vi "Main.vi"() -> ()   [LabVIEW 2026]
doc: "This template is for the Queued Message Handler design pattern.\n\nThe Event Handling Loop generates messages based on user interface actions.\n\nThe Message Handling Loop processes messages generated by the Event Handling Loop, or by other messages. The messages are string values, so new messages can be added easily to the Message Cases case structure in the Message Handling Loop. Each message cluster can also provide an optional value for Message Data, which is a variant that can be converted to whatever message-specific data is required."
uses:
  controls/Controls.ctl
  controls/Program_Settings.ctl
  controls/Display_Panel.ctl
  controls/UI Data.ctl
  support/Message Queue/Enqueue Message (Single).vi
  <vilib>/Utility/error.llb/Error Cluster From Error Code.vi
  <vilib>/ErrorRing/Error Ring.xnode
  support/Message Queue/Message Queue.lvlib
  support/User Event - Stop/User Event - Stop.lvlib
panel:
  out "Display Panel":T1 {"Run time" format="%#_4g"}
  in  "Cluster":T2
  in  "Controls":T3 {"Incline" min=0.0 max=10.0 step=1.0 format="%#_2g"; "Speed" min=0.0 max=10.0 step=0.5 format="%#_2g"}
  in  "Exit":bool
  # "Control Panel"
  # "Manual Setting"
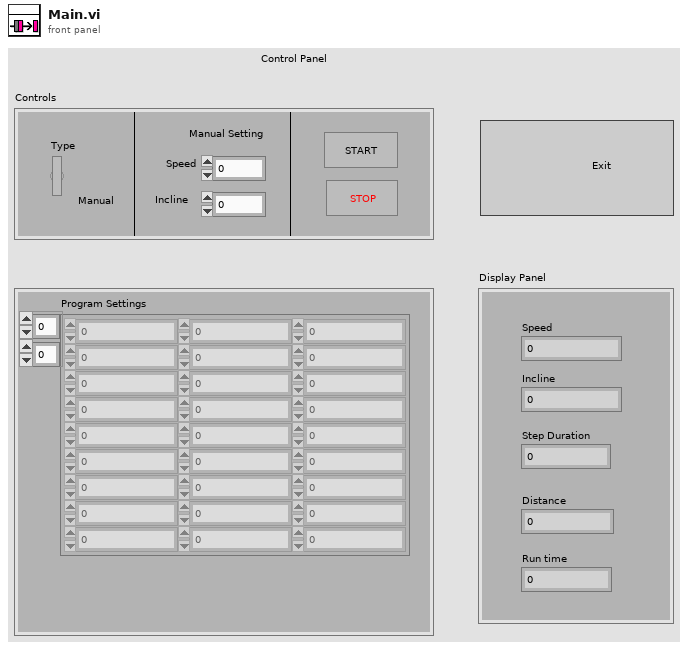
[diagram p1: front panel]
types:
  T1 = typedef "Display_Panel.ctl" = cluster{"Speed":dbl, "Incline":dbl, "Step Duration":dbl, "Distance":dbl, "Run time":dbl}
  T2 = typedef "Program_Settings.ctl" = cluster{"Program Settings":dbl[][]}
  T3 = typedef "Controls.ctl" = cluster{"Type":bool, "Speed":dbl, "Incline":dbl, "Start":bool, "stop":bool}
  T4 = typedef "UI Data.ctl" = cluster{"Boolean":bool, "String":string, "Tick Count":dbl, "Data Display Ref":refnum<vi>, "Exit Button Ref":refnum<vi>, "Display Panel":T1, "Controls":T3, "Controls Ref":refnum<vi>, "Display Panel Ref":refnum<vi>, "Tick Counter":dbl}
  T5 = typedef "Message Queue.lvlib/All Message Queues.ctl" = cluster{"UI":refnum<queue>}
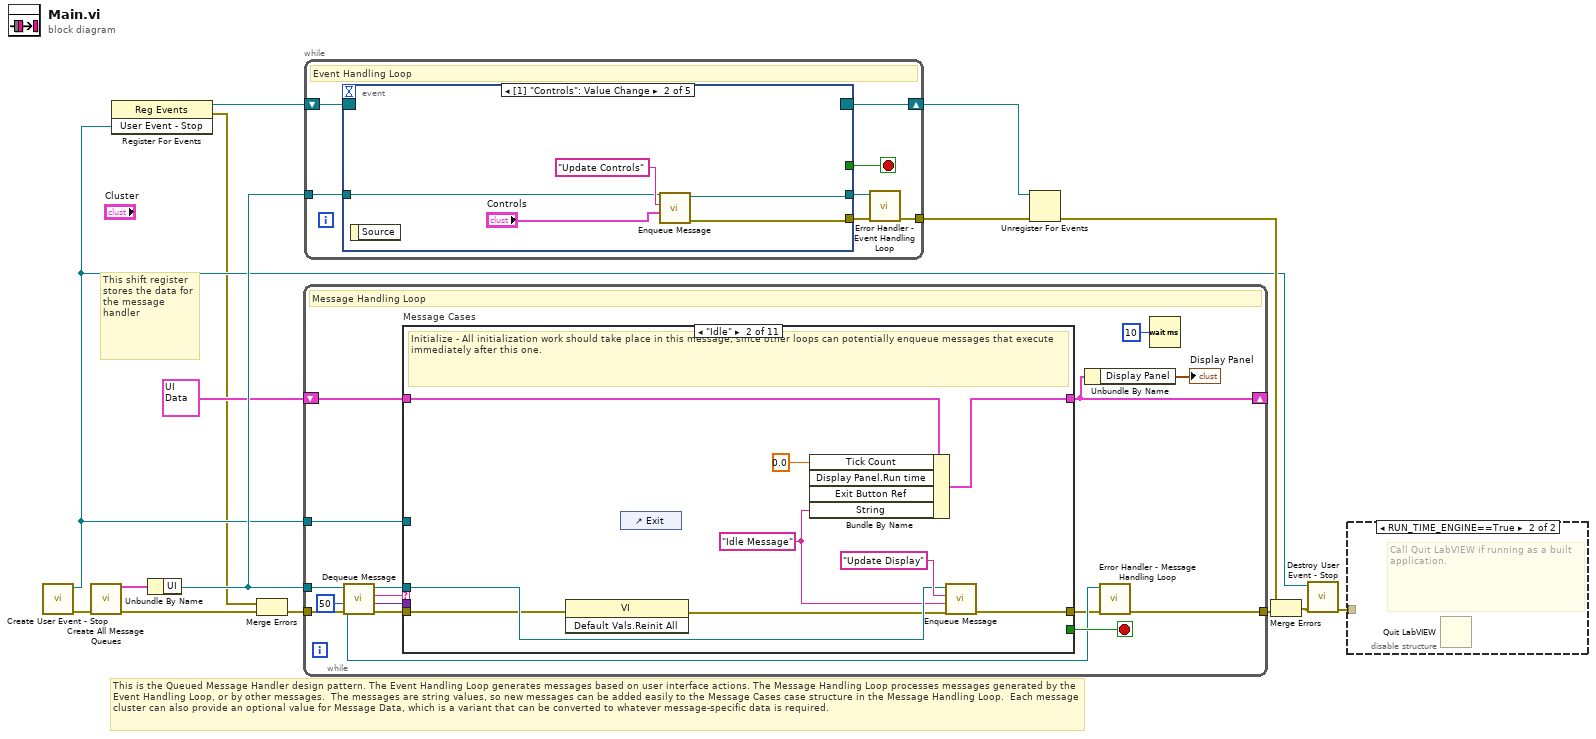
[diagram p0: block diagram]
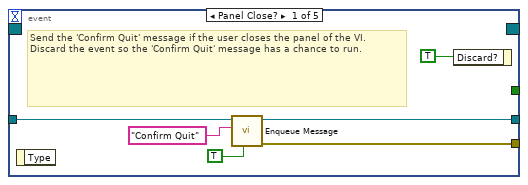
[diagram p3: hidden frame]
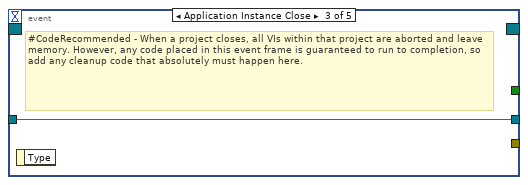
[diagram p4: hidden frame]
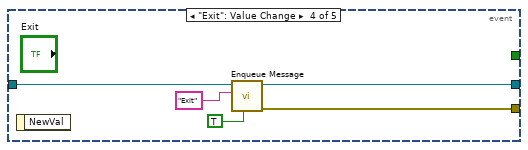
[diagram p5: hidden frame]
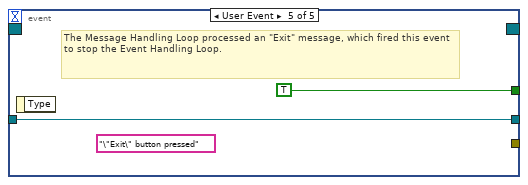
[diagram p6: hidden frame]
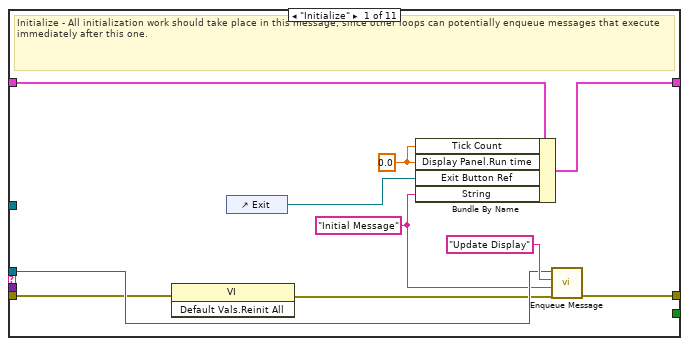
[diagram p7: hidden frame]
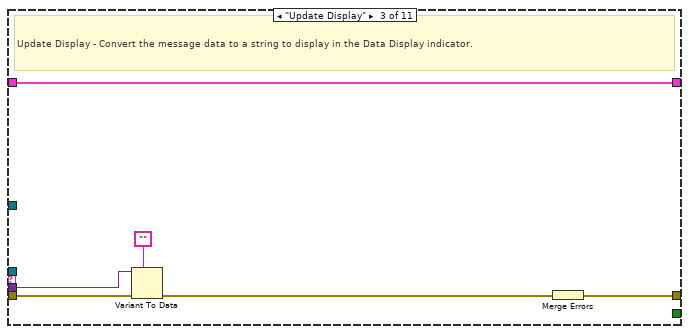
[diagram p8: hidden frame]
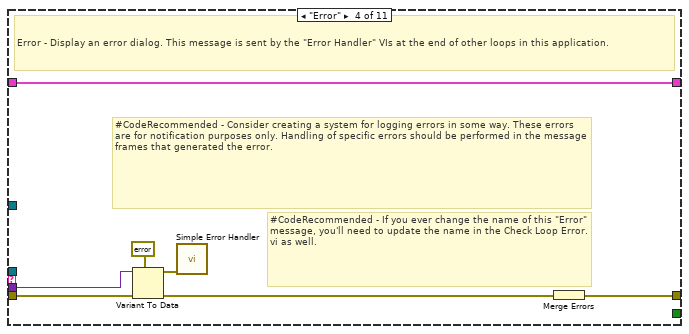
[diagram p9: hidden frame]
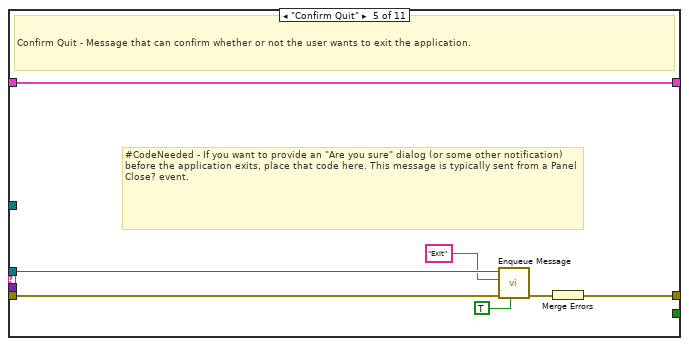
[diagram p10: hidden frame]
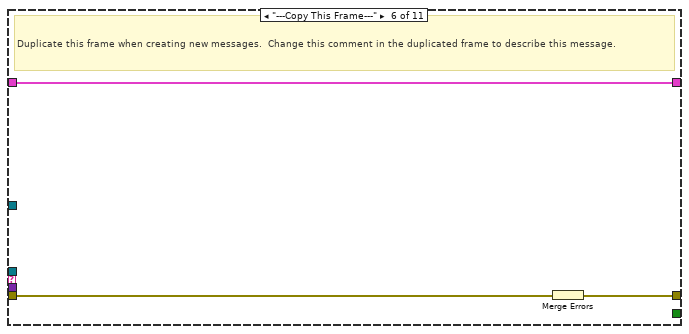
[diagram p11: hidden frame]
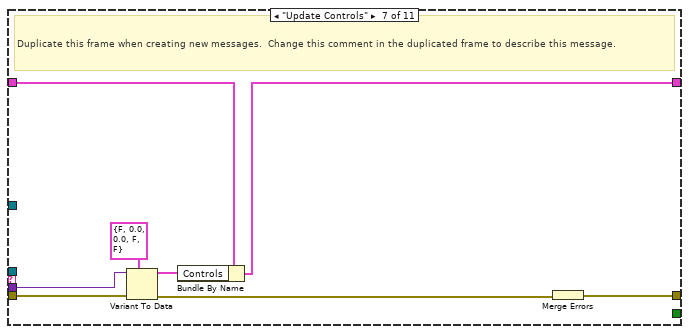
[diagram p12: hidden frame]
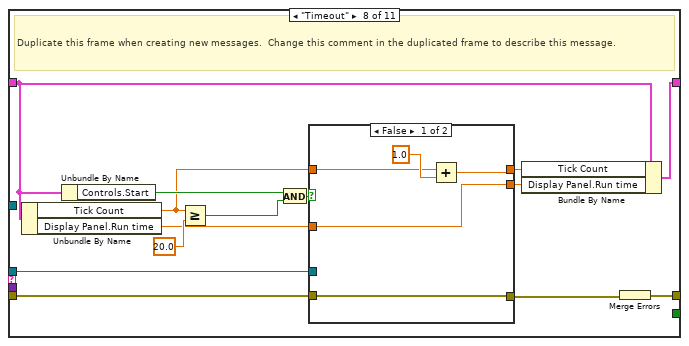
[diagram p13: hidden frame]
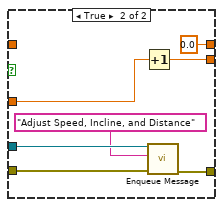
[diagram p14: hidden frame]
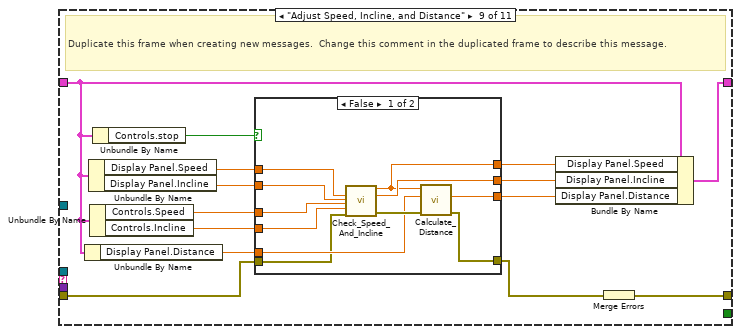
[diagram p15: hidden frame]
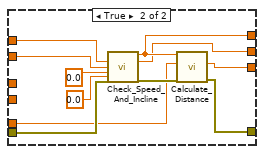
[diagram p16: hidden frame]
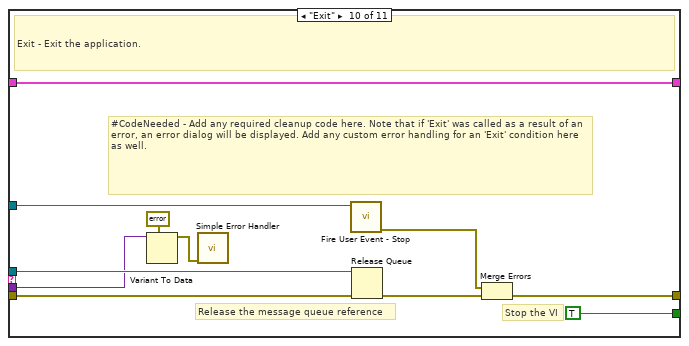
[diagram p17: hidden frame]
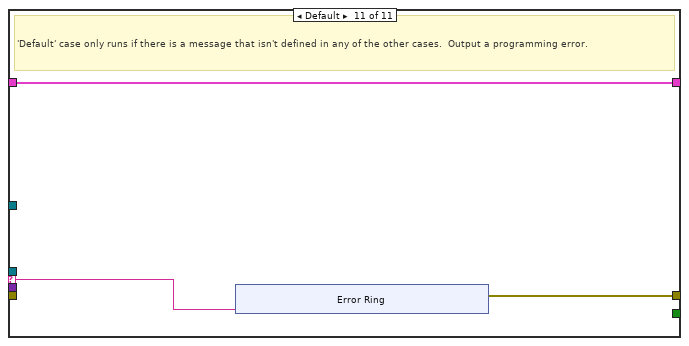
[diagram p18: hidden frame]
diagram:
  # "This is the Queued Message Handler design pattern. The Event Handling Loop generates messages based on user interface actions. The Message Handling Loop processes messages generated by the Event Handling Loop, or by other messages.  The messages are string values, so new messages can be added easily to the Message Cases case structure in the Message Handling Loop.  Each message cluster can also provide an optional value for Message Data, which is a variant that can be converted to whatever message-specific data is required."
  # "This shift register stores the data for the message handler"
  n1 = call "Create User Event - Stop.vi"() -> ("error out"=w11:errorcluster, "User Event - Stop"=w3:refnum<user-event>)  [unwired: 10 in]
  n2 = call "Create All Message Queues.vi"("error in (no error)"=w11) -> ("error out"=w15:errorcluster, "Message Queues out"=w14:T5)  [unwired: 9 in]
  n3 = register-events(w3) -> (reference out=w4:refnum<event-registration>, error out=w1:errorcluster)  [unwired: 2 in]
  n4 = Unbundle By Name(w14) -> ("UI"=w12:refnum<queue>)
  n5 = Merge Errors(w1, w15) -> (w2:errorcluster)
  n6 = while {
    tunnel: w12 -> [w23]
    shift-right: [w19] -> _
    shift-left: T4 {"Boolean"=FALSE, "String"="", "Tick Count"=0.0, "Data Display Ref"=refnum, "Exit Button Ref"=refnum, "Display Panel"={"Speed"=0.0, "Incline"=0.0, "Step Duration"=0.0, "Distance"=0.0, "Run time"=0.0}, "Controls"={"Type"=FALSE, "Speed"=0.0, "Incline"=0.0, "Start"=FALSE, "stop"=FALSE}, "Controls Ref"=refnum, "Display Panel Ref"=refnum, "Tick Counter"=0.0} ("Data Cluster") -> [w30]
    tunnel: w3 -> [w28]
    tunnel: w2 -> [w27]
    tunnel: [w21] -> w13
    stop <- w29 stop-if-true
    # "Message Handling Loop"
    n7 = call "Dequeue Message.vi"("error in (no error)"=w27, "timeout in ms (-1)"=50, "Message Queue"=w23) -> ("error out"=w26:errorcluster, "Message Data"=w24:variant, "Message"=w25:string, "dup Message Queue"=w22:refnum<queue>)  [unwired: 5 in]
    n8 = case "Message Cases" shown="\"Idle\"" w25 {
      selector: w25 -> [_ _ _ _ _ _ _ _ _ _ w154]
      tunnel: w22 -> [w35 w45 _ _ w65 _ _ w90 _ w153 _]
      tunnel: w26 -> [w33 w43 w53 w62 w69 w72 w79 w92 w113 w146 _]
      tunnel: [w40 w49 w54 w56 w67 w70 w80 w94 w120 w149 w155] -> w20
      tunnel: w30 -> [w39 w48 w55 w61 w68 w71 w75 w89 w109 w152 w156]
      tunnel: [w38 w47 w55 w61 w68 w71 w73 w93 w119 w152 w156] -> w19
      tunnel: [_ _ _ _ _ _ _ _ _ TRUE _] -> w29
      tunnel: w24 -> [_ _ w52 w60 _ _ w77 _ _ w143 _]
      tunnel: w28 -> [_ _ _ _ _ _ _ _ _ w148 _]
      frame "Initialize" {
        w31 = 0.0 ("Total Time")
        w34 = "Initial Message" ("Initial Message")
        # "Initialize - All initialization work should take place in this message, since other loops can potentially enqueue messages that execute immediately after this one."
        n9 = invoke class="VI" method="Default Vals.Reinit All"(error in=w33) -> (error out=w32:errorcluster)  [unwired: 2 in, 2 out]
        n10 = control-ref of="Exit"() -> (w37:refnum<vi>)
        n11 = Bundle By Name(cluster=w39, "Tick Count"=w31, "Display Panel.Run time"=w31, "Exit Button Ref"=w37, "String"=w34) -> (w38:T4)
        n12 = call-poly "Enqueue Message.vi"("error in (no error)"=w32, "Message Data"=w34, "Message"="Update Display", "Message Queue"=w35) -> ("error out"=w40:errorcluster)  [unwired: 6 in, 1 out]
      }
      frame "Idle" {
        w44 = "Idle Message" ("Initial Message")
        # "Initialize - All initialization work should take place in this message, since other loops can potentially enqueue messages that execute immediately after this one."
        n13 = invoke class="VI" method="Default Vals.Reinit All"(error in=w43) -> (error out=w42:errorcluster)  [unwired: 2 in, 2 out]
        n14 = control-ref of="Exit"() -> ()  [unwired: 1 out]
        n15 = Bundle By Name(cluster=w48, "Tick Count"=0.0 ("Total Time"), "String"=w44) -> (w47:T4)  [unwired: 2 in]
        n16 = call-poly "Enqueue Message.vi"("error in (no error)"=w42, "Message Data"=w44, "Message"="Update Display", "Message Queue"=w45) -> ("error out"=w49:errorcluster)  [unwired: 6 in, 1 out]
      }
      frame "Update Display" {
        # "Update Display - Convert the message data to a string to display in the Data Display indicator."
        n17 = Variant To Data(error in=w53, type="", Variant=w52) -> (error out=w50:errorcluster)  [unwired: 1 out]
        n18 = Merge Errors(w50) -> (w54:errorcluster)
      }
      frame "Error" {
        # "#CodeRecommended - If you ever change the name of this \"Error\" message, you'll need to update the name in the Check Loop Error.vi as well."
        # "#CodeRecommended - Consider creating a system for logging errors in some way. These errors are for notification purposes only. Handling of specific errors should be performed in the message frames that generated the error."
        # "Error - Display an error dialog. This message is sent by the \"Error Handler\" VIs at the end of other loops in this application."
        n19 = Variant To Data(error in=w62, type=errorcluster {"status"=FALSE, "code"=0, "source"=""} ("error constant"), Variant=w60) -> (data=w58:errorcluster, error out=w57:errorcluster)
        n20 = call <vilib>:"Simple Error Handler.vi"("error in (no error)"=w58) -> ()  [unwired: 4 in, 5 out]
        n21 = Merge Errors(w57) -> (w56:errorcluster)
      }
      frame "Confirm Quit" {
        # "#CodeNeeded - If you want to provide an \"Are you sure\" dialog (or some other notification) before the application exits, place that code here. This message is typically sent from a Panel Close? event."
        # "Confirm Quit - Message that can confirm whether or not the user wants to exit the application."
        n22 = call-poly "Enqueue Message.vi"("Priority Message? (F)"=TRUE, "error in (no error)"=w69, "Message"="Exit", "Message Queue"=w65) -> ("error out"=w66:errorcluster)  [unwired: 6 in, 1 out]
        n23 = Merge Errors(w66) -> (w67:errorcluster)
      }
      frame "---Copy This Frame---" {
        # "Duplicate this frame when creating new messages.  Change this comment in the duplicated frame to describe this message."
        n24 = Merge Errors(w72) -> (w70:errorcluster)
      }
      frame "Update Controls" {
        # "Duplicate this frame when creating new messages.  Change this comment in the duplicated frame to describe this message."
        n25 = Variant To Data(error in=w79, type=T3 {"Type"=FALSE, "Speed"=0.0, "Incline"=0.0, "Start"=FALSE, "stop"=FALSE} ("Controls"), Variant=w77) -> (data=w74:T3, error out=w78:errorcluster)
        n26 = Bundle By Name(cluster=w75, "Controls"=w74) -> (w73:T4)
        n27 = Merge Errors(w78) -> (w80:errorcluster)
      }
      frame "Timeout" {
        # "Duplicate this frame when creating new messages.  Change this comment in the duplicated frame to describe this message."
        n28 = Unbundle By Name(w89) -> ("Tick Count"=w84:dbl, "Display Panel.Run time"=w81:dbl)
        n29 = Unbundle By Name(w89) -> ("Controls.Start"=w88:bool)
        n30 = Greater Or Equal?(x=w84, y=20.0) -> (x >= y?=w82:bool)
        n31 = And(x=w88, y=w82) -> (x .and. y?=w87:bool)
        n32 = case shown="False" w87 {
          tunnel: w92 -> [w99 w106]
          tunnel: [w99 w105] -> w91
          tunnel: w90 -> [_ w104]
          tunnel: w84 -> [w96 _]
          tunnel: [w95 w101] -> w86
          tunnel: [w97 0.0] -> w85
          tunnel: w81 -> [w95 w100]
          frame False {
            n33 = Add(x=w96, y=1.0) -> (x+y=w97:dbl)
          }
          frame True {
            n34 = Increment(x=w100) -> (x+1=w101:dbl)
            n35 = call-poly "Enqueue Message.vi"("error in (no error)"=w106, "Message"="Adjust Speed, Incline, and Distance", "Message Queue"=w104) -> ("error out"=w105:errorcluster)  [unwired: 7 in, 1 out]
          }
        }
        n36 = Bundle By Name(cluster=w89, "Tick Count"=w85, "Display Panel.Run time"=w86) -> (w93:T4)
        n37 = Merge Errors(w91) -> (w94:errorcluster)
      }
      frame "Adjust Speed, Incline, and Distance" {
        # "Duplicate this frame when creating new messages.  Change this comment in the duplicated frame to describe this message."
        n38 = Unbundle By Name(w109) -> ("Display Panel.Distance"=w112:dbl)
        n39 = Unbundle By Name(w109) -> ("Display Panel.Speed"=w116:dbl, "Display Panel.Incline"=w118:dbl)
        n40 = Unbundle By Name(w109) -> ("Controls.Speed"=w111:dbl, "Controls.Incline"=w117:dbl)
        n41 = Unbundle By Name(w109) -> ("Controls.stop"=w108:bool)
        n42 = case shown="False" w108 {
          tunnel: w118 -> [w131 w139]
          tunnel: w117 -> [w130 _]
          tunnel: w116 -> [w122 w138]
          tunnel: [w121 w133] -> w115
          tunnel: [w129 w132] -> w114
          tunnel: w113 -> [w124 w142]
          tunnel: w112 -> [w127 w134]
          tunnel: w111 -> [w126 _]
          tunnel: [w125 w135] -> w110
          tunnel: [w123 w136] -> w107
          frame False {
            n43 = call "Check_Speed_And_Incline.vi"("Display Speed"=w122, "Display Incline"=w131, "Control Speed"=w126, "Control Incline"=w130, "error in (no error)"=w124) -> ("Speed"=w121:dbl, "Incline"=w129:dbl, "error out"=w128:errorcluster)  [unwired: 8 in]
            n44 = call "Calculate_Distance.vi"("Speed"=w121, "Current Distance"=w127, "error in (no error)"=w128) -> ("New Distance"=w125:dbl, "error out"=w123:errorcluster)  [unwired: 6 in]
          }
          frame True {
            n45 = call "Check_Speed_And_Incline.vi"("Display Speed"=w138, "Display Incline"=w139, "Control Speed"=0.0 ("Total Time"), "Control Incline"=0.0 ("Display Incline"), "error in (no error)"=w142) -> ("Speed"=w133:dbl, "Incline"=w132:dbl, "error out"=w137:errorcluster)  [unwired: 8 in]
            n46 = call "Calculate_Distance.vi"("Speed"=w133, "Current Distance"=w134, "error in (no error)"=w137) -> ("New Distance"=w135:dbl, "error out"=w136:errorcluster)  [unwired: 6 in]
          }
        }
        n47 = Bundle By Name(cluster=w109, "Display Panel.Speed"=w115, "Display Panel.Incline"=w114, "Display Panel.Distance"=w110) -> (w119:T4)
        n48 = Merge Errors(w107) -> (w120:errorcluster)
      }
      frame "Exit" {
        # "Stop the VI"
        # "Release the message queue reference"
        # "#CodeNeeded - Add any required cleanup code here. Note that if 'Exit' was called as a result of an error, an error dialog will be displayed. Add any custom error handling for an 'Exit' condition here as well."
        # "Exit - Exit the application."
        n49 = Variant To Data(type=errorcluster {"status"=FALSE, "code"=0, "source"=""} ("error constant"), Variant=w143) -> (data=w144:errorcluster)  [unwired: 1 in, 1 out]
        n50 = call <vilib>:"Simple Error Handler.vi"("error in (no error)"=w144) -> ()  [unwired: 4 in, 5 out]
        n51 = call "Fire User Event - Stop.vi"("User Event - Stop"=w148) -> ("error out"=w147:errorcluster)  [unwired: 10 in]
        n52 = Release Queue(queue=w153, error in (no error)=w146) -> (error out=w150:errorcluster)  [unwired: 1 in, 2 out]
        n53 = Merge Errors(w147, w150) -> (w149:errorcluster)
      }
      frame Default {
        # "'Default' case only runs if there is a message that isn't defined in any of the other cases.  Output a programming error."
        n54 = xnode "Error Ring"("parameter 0"=w154) -> ("error out"=w155:errorcluster)
      }
    }
    n55 = Unbundle By Name(w19) -> ("Display Panel"=→"Display Panel":T1)
    n56 = call "Error Handler - Message Handling Loop.vi"("error in (no error)"=w20, "Message Queue"=w22) -> ("dup error in"=w21:errorcluster)  [unwired: 8 in, 1 out]
    n57 = Wait (ms)(milliseconds to wait=u32 10) -> ()  [unwired: 1 out]
  }
  n58 = while {
    tunnel: w12 -> [w170]
    shift-right: [w168] -> w8
    shift-left: w4 -> [w169]
    tunnel: [w164] -> w5
    stop <- w166 stop-if-true
    # "Event Handling Loop"
    n59 = event shown="[1] \"Controls\": Value Change" {
      selector: w169 -> [_ _ _ _ _]
      dyn-events: [_ _ _ _ _] -> w168
      timeout: _ -> [_ _ _ _ _]
      tunnel: [_ _ _ _ TRUE ("Discard?")] -> w166
      tunnel: w170 -> [w175 w180 w182 w187 w189]
      tunnel: [w174 w178 _ w186 _] -> w167
      tunnel: [w173 w179 w182 w185 w189] -> w165
      event Panel Close? {
        # "Send the 'Confirm Quit' message if the user closes the panel of the VI. Discard the event so the 'Confirm Quit' message has a chance to run."
        n60 = event-data() -> ()  [unwired: 1 in, 1 out]
        n61 = call-poly "Enqueue Message.vi"("Priority Message? (F)"=TRUE, "Message"="Confirm Quit", "Message Queue"=w175) -> ("error out"=w174:errorcluster, "dup Message Queue"=w173:refnum<queue>)  [unwired: 7 in]
        n62 = event-data("Discard?"=TRUE) -> ()  [unwired: 1 in, 1 out]
      }
      event Value Change {
        n63 = event-data() -> ()  [unwired: 1 in, 1 out]
        n64 = call-poly "Enqueue Message.vi"("Message Data"="Controls", "Message"="Update Controls", "Message Queue"=w180) -> ("error out"=w178:errorcluster, "dup Message Queue"=w179:refnum<queue>)  [unwired: 7 in]
      }
      event Application Instance Close {
        # "#CodeRecommended - When a project closes, all VIs within that project are aborted and leave memory. However, any code placed in this event frame is guaranteed to run to completion, so add any cleanup code that absolutely must happen here."
        n65 = event-data() -> ()  [unwired: 1 in, 1 out]
      }
      event "Exit": Value Change {
        n66 = event-data() -> ()  [unwired: 1 in, 1 out]
        n67 = call-poly "Enqueue Message.vi"("Priority Message? (F)"=TRUE, "Message"="Exit", "Message Queue"=w187) -> ("error out"=w186:errorcluster, "dup Message Queue"=w185:refnum<queue>)  [unwired: 7 in]
      }
      event User Event {
        (unwired) "\"Exit\" button pressed" ("VI Stopped")
        # "The Message Handling Loop processed an \"Exit\" message, which fired this event to stop the Event Handling Loop."
        n68 = event-data() -> ()  [unwired: 1 in, 1 out]
      }
    }
    n69 = call "Error Handler - Event Handling Loop.vi"("error in (no error)"=w167, "Message Queue"=w165) -> ("dup error in"=w164:errorcluster)  [unwired: 8 in, 1 out]
  }
  n70 = Unregister For Events(event registration refnum=w8, error in=w5) -> (error out=w9:errorcluster)
  n71 = Merge Errors(w9, w13) -> (w10:errorcluster)
  n72 = call "Destroy User Event - Stop.vi"("error in (no error)"=w10, "User Event - Stop"=w3) -> ("error out"=w6:errorcluster)  [unwired: 9 in]
  n73 = disable-structure shown="RUN_TIME_ENGINE==True" {
    disable-tunnel: w6 -> [_ _]
    frame condition #0 (active) {
    }
    frame condition #1 {
      # "Call Quit LabVIEW if running as a built application."
      n74 = Quit LabVIEW() -> ()  [unwired: 1 in]
    }
  }
